vi "Get-full-file-path.vi"(8 "error in (no error)":errorcluster, 10 "Dialog?":bool, 11 "SettingsFile in":refnum<class "SettingsFile.lvclass">) -> (0 "error out":errorcluster, 1 "Cancelled?":bool, 2 "Full path":path, 3 "SettingsFile out":refnum<class "SettingsFile.lvclass">)   [LabVIEW 2013, in "SettingsFile.lvlib" / "SettingsFile.lvclass"]
uses:
  SettingsFile.lvclass
  SettingsFile.lvclass/SettingsFile.ctl
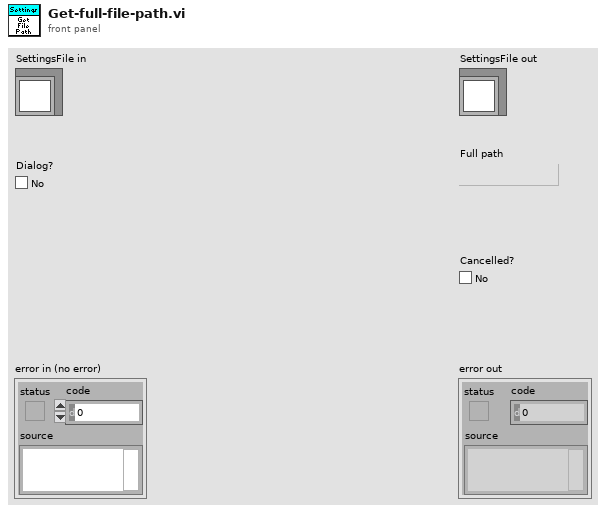
[diagram p1: front panel]
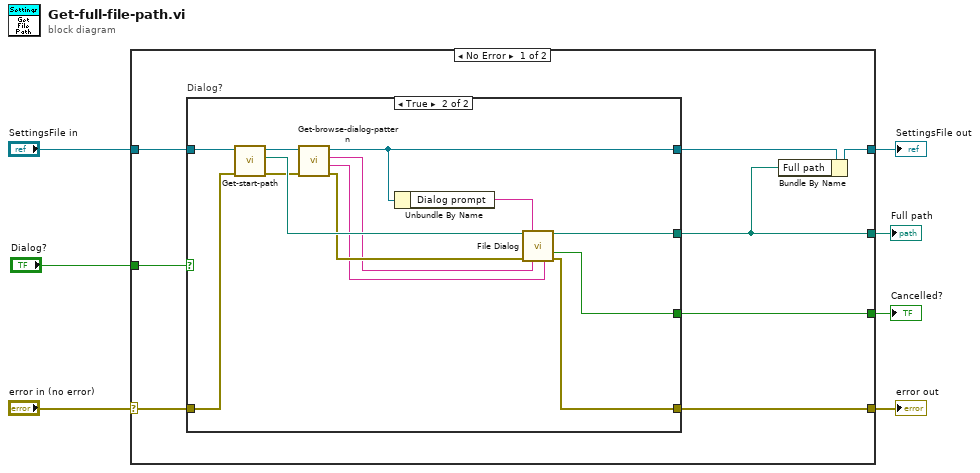
[diagram p0: block diagram]
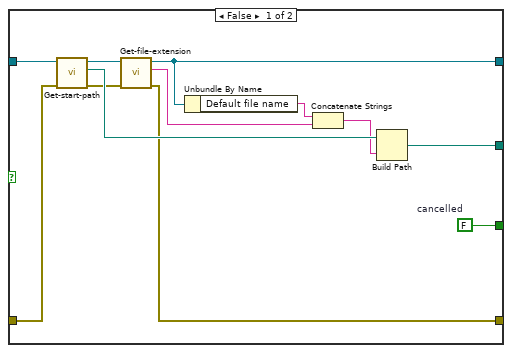
[diagram p2: hidden frame]
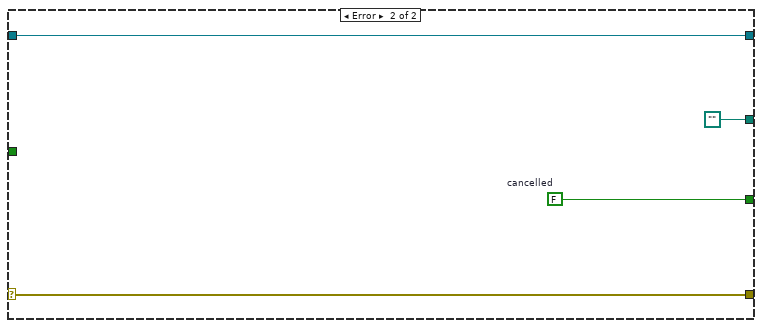
[diagram p3: hidden frame]
diagram:
  n1 = case shown="No Error" "error in (no error)" {
    selector: "error in (no error)" -> [w13 w44]
    tunnel: [w10 w44] -> w6
    tunnel: [w9 w43] -> w4
    tunnel: "SettingsFile in" -> [w15 w43]
    tunnel: "Dialog?" -> [w14 _]
    tunnel: [w8 path ""] -> w2
    tunnel: [w11 w41] -> w1
    frame No Error {
      n2 = case "Dialog?" shown="True" w14 {
        tunnel: w15 -> [w27 w40]
        tunnel: w13 -> [w26 w39]
        tunnel: [w17 w32] -> w12
        tunnel: [w20 w30] -> w8
        tunnel: [w16 w29] -> w11
        tunnel: [w18 w28] -> w10
        frame False {
          w16 = FALSE  # cancelled
          n3 = call "Get-start-path.vi"("error in (no error)"=w26, "SettingsFile in"=w27) -> ("error out"=w19:errorcluster, "File path"=w24:path, "SettingsFile out"=w25:refnum<class "SettingsFile.lvclass">)  [unwired: 7 in]
          n4 = call "Get-file-extension.vi"("error in (no error)"=w19, "SettingsFile in"=w25) -> ("error out"=w18:errorcluster, "File extension"=w22:string, "SettingsFile out"=w17:refnum<class "SettingsFile.lvclass">)  [unwired: 7 in]
          n5 = Unbundle By Name(w17) -> ("Default file name"=w23:string)
          n6 = Concatenate Strings(w23, w22) -> (w21:string)
          n7 = Build Path(base path=w24, name or relative path=w21) -> (appended path=w20:path)
        }
        frame True {
          n8 = call "Get-start-path.vi"("error in (no error)"=w39, "SettingsFile in"=w40) -> ("error out"=w37:errorcluster, "File path"=w38:path, "SettingsFile out"=w36:refnum<class "SettingsFile.lvclass">)  [unwired: 7 in]
          n9 = call "Get-browse-dialog-pattern.vi"("error in (no error)"=w37, "SettingsFile in"=w36) -> ("error out"=w35:errorcluster, "Pattern label"=w33:string, "Pattern"=w34:string, "SettingsFile out"=w32:refnum<class "SettingsFile.lvclass">)  [unwired: 6 in]
          n10 = Unbundle By Name(w32) -> ("Dialog prompt"=w31:string)
          n11 = call "File Dialog"("start path"=w38, "prompt"=w31, "error in"=w35, "pattern (all files)"=w34, "pattern label"=w33) -> ("selected path"=w30:path, "cancelled"=w29:bool, "error out"=w28:errorcluster)  [unwired: 7 in, 1 out]
        }
      }
      n12 = Bundle By Name(cluster=w12, "Full path"=w8) -> (w9:refnum<class "SettingsFile.lvclass">)
    }
    frame Error {
      w41 = FALSE  # cancelled
    }
  }
  "error out" <- w6
  "SettingsFile out" <- w4
  "Full path" <- w2
  "Cancelled?" <- w1
